vi "Write Stiffness Data.vi"(10 "Stiffness Data":T1={"Constrained Displacement"=1.0, "Stiffness"=0.0} {"Constrained Displacement" min=1.0 max=300.0 format="%.1f"; "Stiffness" format="%#.3f"}, 11 "StiffnessLog in":refnum<class "StiffnessLog.lvclass">) -> (3 "StiffnessLog out":refnum<class "StiffnessLog.lvclass">)   [LabVIEW 2013, in "StiffnessLog.lvclass"]
uses:
  StiffnessLog.lvclass
  Typedefs/StiffnessData.ctl
  StiffnessLog.lvclass/StiffnessLog.ctl
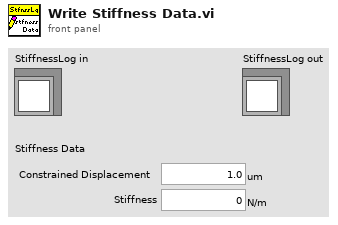
[diagram p1: front panel]
types:
  T1 = typedef "StiffnessData.ctl" = cluster{"Constrained Displacement":dbl[unit], "Stiffness":dbl[unit]}
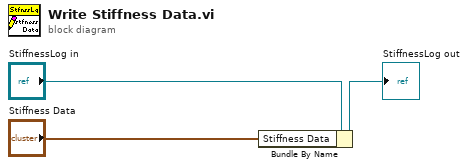
[diagram p0: block diagram]
diagram:
  n1 = Bundle By Name(cluster="StiffnessLog in", "Stiffness Data"="Stiffness Data") -> (→"StiffnessLog out":refnum<class "StiffnessLog.lvclass">)
